vi "struct_abs_mix_dp_dT_Tx.vi"(0 "Reference working pair (Input)":i64, 5 "Temperature in K (Input)":dbl, 7 "Mole fraction in liquid phase in mol/mol (Input)":dbl, 11 "Error (Input)":errorcluster) -> (4 "Der. of equilibrium pressure wrt temperature in Pa/K (Output)":dbl, 15 "Error (Output)":errorcluster)   [LabVIEW 2017]
doc: "abs_mix_dp_dT_Tx:\n * -----------------\n *\n * Calculates derivative of equilibrium pressure with respect to temperature in\n * Pa/K depending on temperature T_K in K and mole fraction in liquid phase\n * x_molmol in mol/mol.\n *\n * Parameters:\n * -----------\n * double T_K:\n * Equilibrium temperature in K.\n * double x_1_molmol:\n * Equilibrium mole fraction in liquid phase in mol/mol.\n * struct *WorkingPair:\n * Pointer of WorkingPair-struct.\n *\n * Returns:\n * --------\n * double:\n * Derivative of equilibrium pressure wrt temperature in Pa/K.\n *\n * Remarks:\n * --------\n * This function is only valid for isotherm models based on mixing rules.\n * Derivative is calculated numerically by the symmetric derivative using\n * h = 0.0001 K as small change.\n *\n * History: \n * --------\n * 07/14/2021, by Jannik Driesel (supervised by Mirko Engelpracht):\n * First implementation."
uses:
  data/win32bit/libsorpPropLib.dll
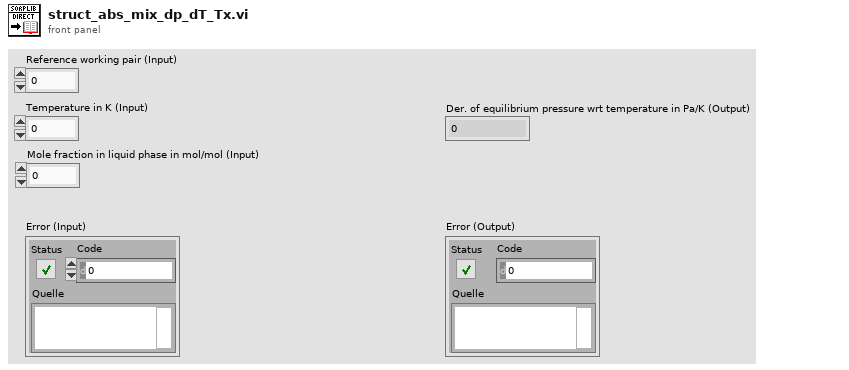
[diagram p1: front panel]
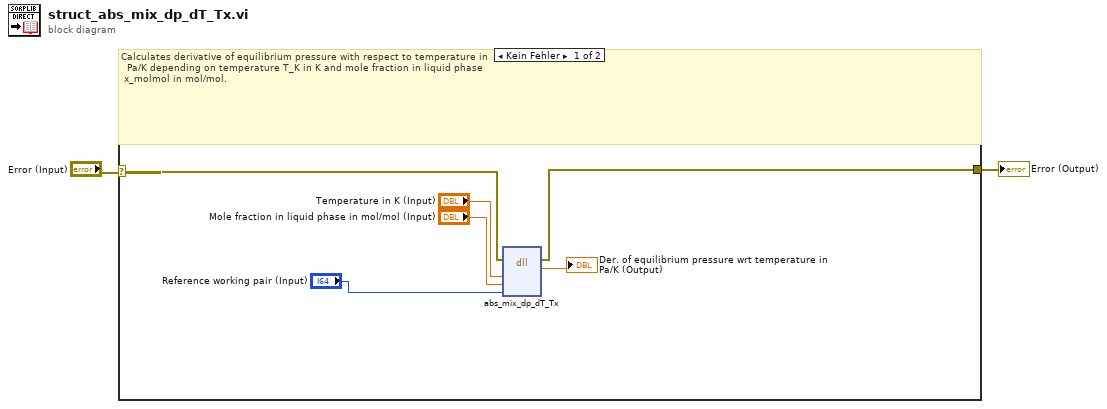
[diagram p0: block diagram]
diagram:
  n1 = case shown="Kein Fehler" "Error (Input)" {
    selector: "Error (Input)" -> [w8 w9]
    tunnel: [w7 w9] -> w2
    frame No Error {
      # "Calculates derivative of equilibrium pressure with respect to temperature in\n  Pa/K depending on temperature T_K in K and mole fraction in liquid phase\n x_molmol in mol/mol."
      n2 = dll-call lib="D:/Driesel/SorpLibLocal/LabVIEW_wrapper/data/win32bit/libsorpPropLib.dll" fn="abs_mix_dp_dT_Tx"(error in=w8, "T_K"="Temperature in K (Input)", "x_1_molmol"="Mole fraction in liquid phase in mol/mol (Input)", "workingPair"="Reference working pair (Input)") -> (error out=w7:errorcluster, "dp_dT_PaK"=→"Der. of equilibrium pressure wrt temperature in Pa/K (Output)":dbl)  [unwired: 5 in, 1 out]
    }
    frame Error {
      # "Error - No calculations"
    }
  }
  "Error (Output)" <- w2
